vi "Get Key Value (Timestamp).vi"(5 "Key name":string, 6 "Default value":timestamp, 7 "Section name":string, 8 "error in (no error)":errorcluster, 11 "Carya Config in":refnum<class "Carya Config.lvclass">) -> (0 "error out":errorcluster, 1 "Found?":bool, 2 "Value":timestamp, 3 "Carya Config out":refnum<class "Carya Config.lvclass">)   [LabVIEW 2013, in "Carya Config.lvclass"]
doc: "Copyright 2018, Carya Automatisering, Wiebe Walstra."
uses:
  Carya Config.lvclass
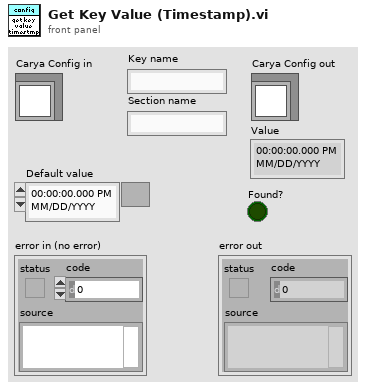
[diagram p1: front panel]
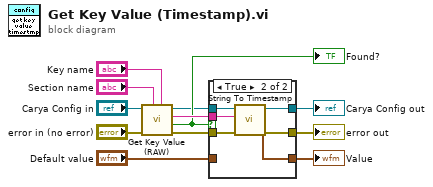
[diagram p0: block diagram]
diagram:
  n1 = call-dynamic "Get Key Value (RAW).vi"("Key name"="Key name", "Section name"="Section name", "error in (no error)"="error in (no error)", "Carya Config in"="Carya Config in") -> ("error out"=w11:errorcluster, "Found?"=w5:bool, "Value"=w6:string, "Carya Config out"=w2:refnum<class "Carya Config.lvclass">)  [unwired: 4 in]
  "Found?" <- w5
  n2 = case shown="True" w5 {
    tunnel: w11 -> [w14 w19]
    tunnel: [w14 w21] -> w7
    tunnel: w6 -> [_ w18]
    tunnel: "Default value" -> [w15 _]
    tunnel: [w15 w20] -> w4
    tunnel: w2 -> [w13 w17]
    tunnel: [w13 w16] -> w1
    frame False {
    }
    frame True {
      n3 = call-dynamic "String To Timestamp.vi"("error in (no error)"=w19, "String"=w18, "Registry Object"=w17) -> ("error out"=w21:errorcluster, "Unescaped string"=w20:timestamp, "Registry Object"=w16:refnum<class "Carya Config.lvclass">)  [unwired: 6 in]
    }
  }
  "error out" <- w7
  "Carya Config out" <- w1
  "Value" <- w4
